vi "Find Scalar Group.vi"(8 "error in (no error)":errorcluster, 10 "Group Name":string, 11 "FPGA Addon refnum in":T1 format="%.0x") -> (0 "error out":errorcluster, 1 "Found ?":bool, 2 "Group Scalar Data":T2 {"Scalar Section ref" format="%.0x"; "Group Section ref" format="%.0x"; "Group Scalar Registers"."Data Type" format="%.0x"}, 3 "FPGA Addon refnum out":T1=18446744073709551615 format="%.0x")   [LabVIEW 2018, in "Scripting API.lvlib"]
uses:
  Scripting API.lvlib
  <vilib>/NI Veristand/Custom Device API/Custom Device Item Ref.ctl
  TypeDefs/Group Scalar Data.ctl
  Addon/Addon Shared/Types/Register Information.ctl
  Addon/Addon Shared/Types/Data Type.ctl
  Addon/Addon Shared/Types/FG Action.ctl
  Addon/Addon Shared/SubVIs/Constants.vi
  <vilib>/NI/NI VeriStand Advanced SysDef API/_SubVIs/SysDef.Search.GUID.vi
  <vilib>/NI/NI VeriStand Advanced SysDef API/SysDef API/SysDef.Property.Get.vi
  <vilib>/NI/NI VeriStand Advanced SysDef API/_SubVIs/SysDef.Property.Get.Variant.vi
  <vilib>/NI/NI VeriStand Advanced SysDef API/SysDef API/SysDef.Property.Set.vi
  <vilib>/NI/NI VeriStand Advanced SysDef API/_SubVIs/SysDef.Property.Set.Variant.vi
  <vilib>/NI/NI VeriStand Advanced SysDef API/_SubVIs/SysDef.Search.Name.vi
  <vilib>/NI/NI VeriStand Advanced SysDef API/SysDef API/Advanced System Definition.lvlib
  Addon/Addon Shared/FPGA Addon Shared.lvlib
  <vilib>/NI Veristand/Custom Device API/Custom Device API.lvlib
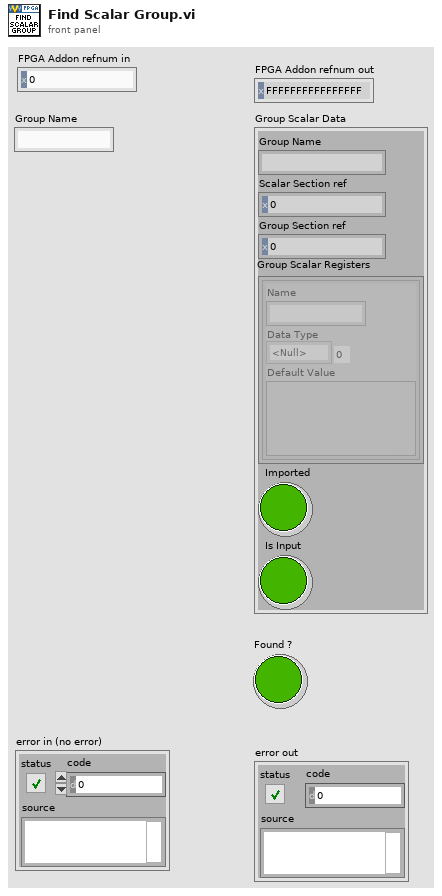
[diagram p1: front panel]
types:
  T1 = typedef "Custom Device API.lvlib/Custom Device Item Ref.ctl" = u64
  T2 = typedef "Scripting API.lvlib/Group Scalar Data.ctl" = cluster{"Group Name":string, "Scalar Section ref":T1, "Group Section ref":T1, "Group Scalar Registers":T3[], "Imported":bool, "Is Input":bool}
  T3 = typedef "FPGA Addon Shared.lvlib/Register Information.ctl" = cluster{"Name":string, "Data Type":T4, "Default Value":variant}
  T4 = typedef "FPGA Addon Shared.lvlib/Data Type.ctl" = enum8{"<Null>", "I8", "I16", "I32", "I64", "U8", "U16", "U32", "U64", "SGL", "Boolean", "Analog PWM In Settings", "Analog PWM In", "Digital PWM In Settings", "Digital PWM In", "Digital PWM Out", "Sine Out", "FXP+/-24.5", "FXP+/-16.5", "FXP+/-32.8", "FXP+/-64.32", "FXP+/-16.7", "FXP+/-20.5", "FXP+/-27.5", "FXP+/-32.16", "FXP+16.3", "FXP+18.3", "Digital Static In", "Digital Static Out", "Digital Static In Settings", "Digital WSS Out", "Quad Encoder Settings", "Quad Encoder In", "Group"}
  T5 = typedef "FPGA Addon Shared.lvlib/FG Action.ctl" = enum8{"GET", "SET"}
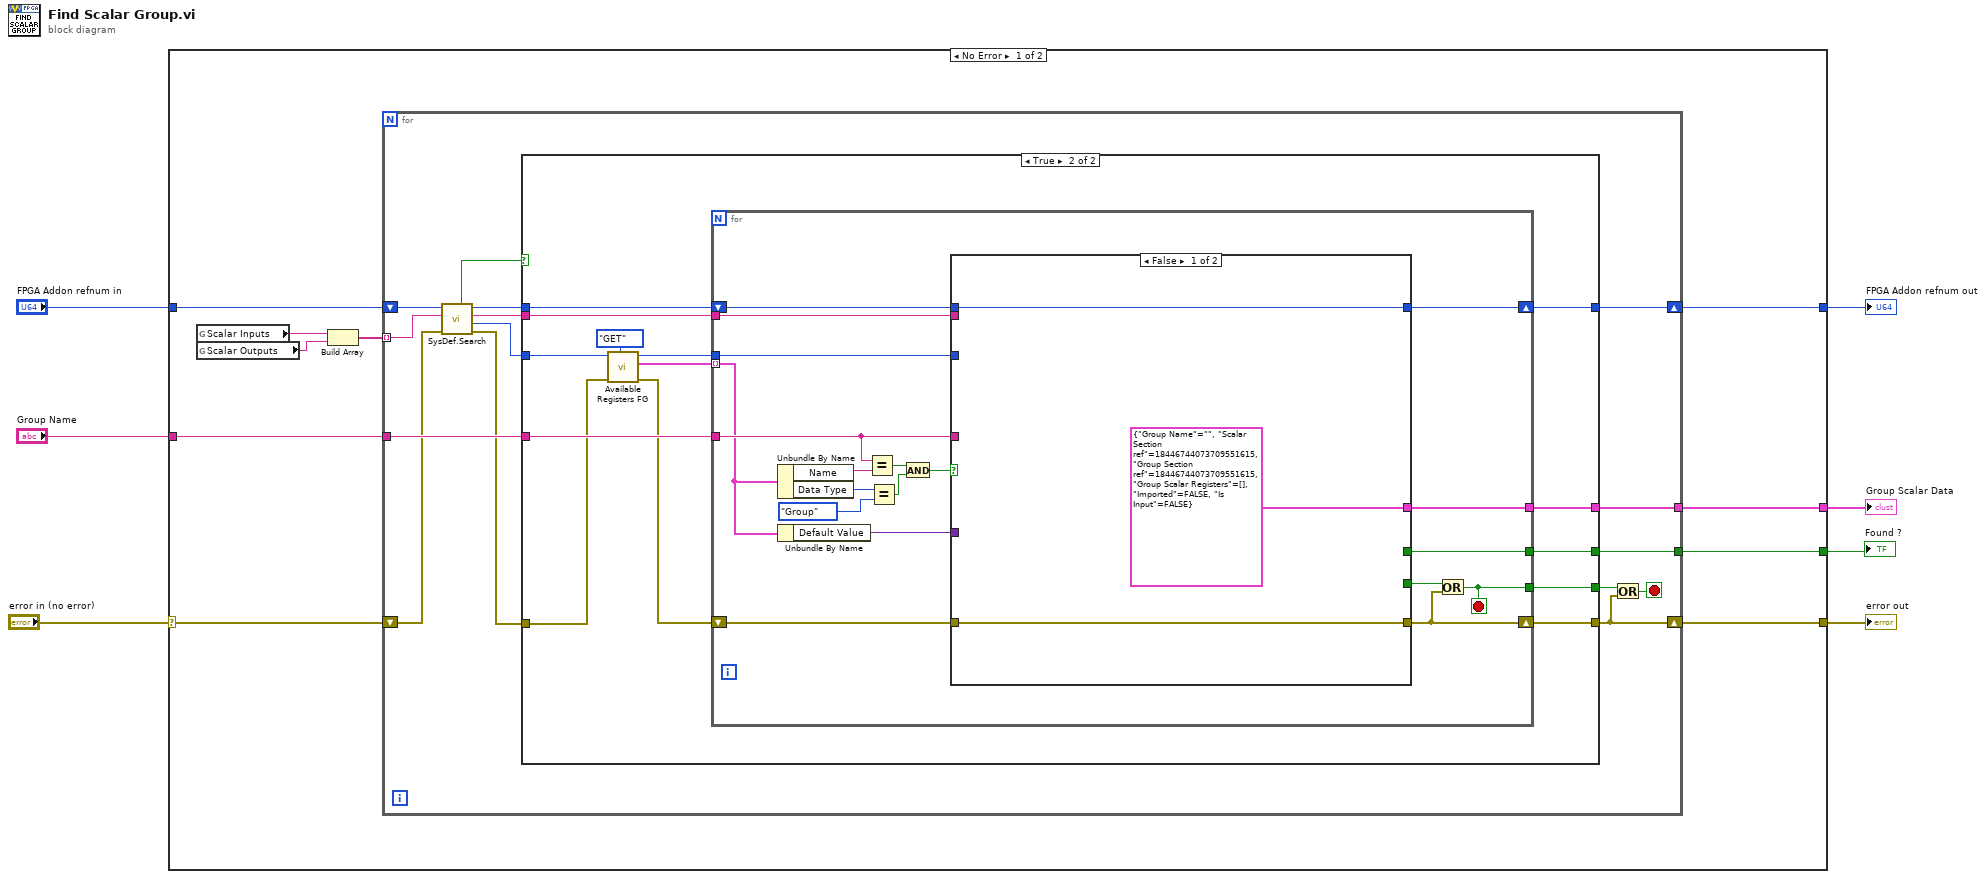
[diagram p0: block diagram]
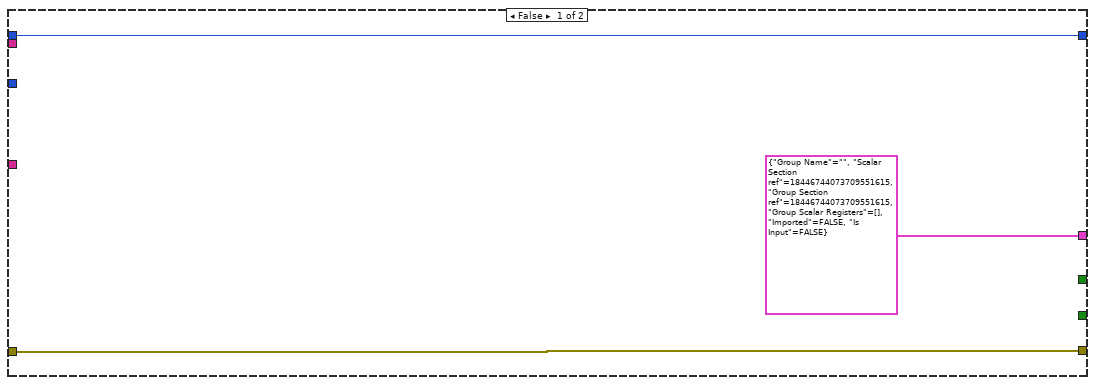
[diagram p2: hidden frame]
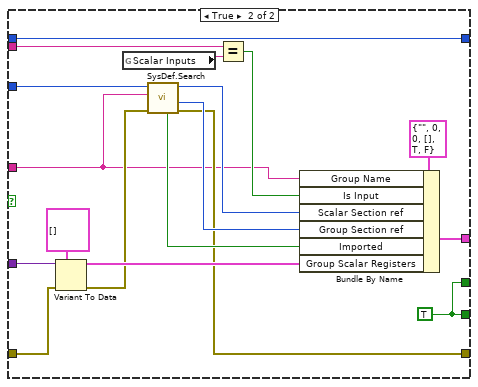
[diagram p3: hidden frame]
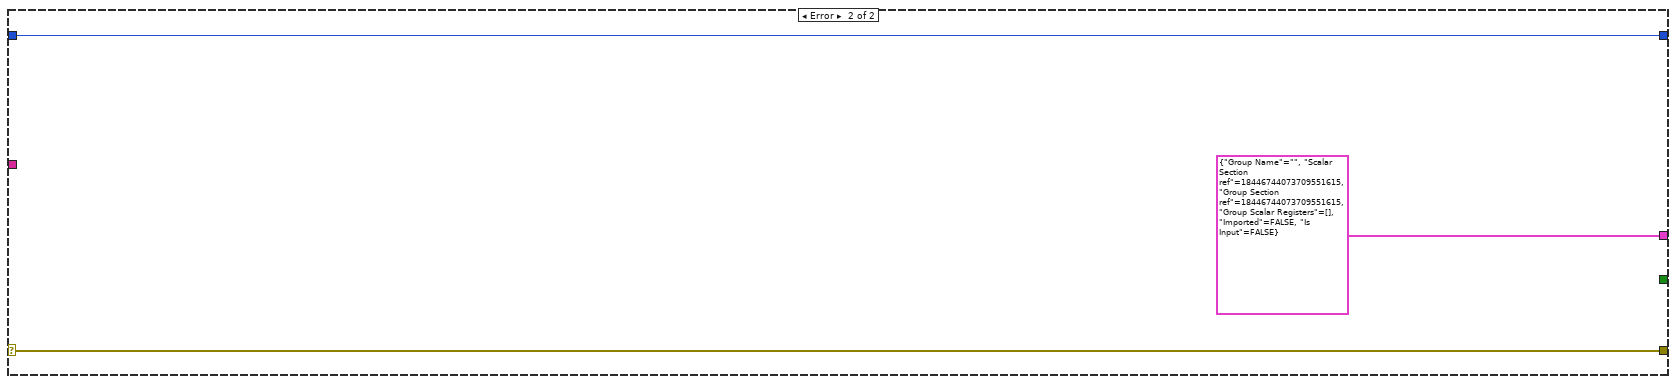
[diagram p4: hidden frame]
diagram:
  n1 = case shown="No Error" "error in (no error)" {
    selector: "error in (no error)" -> [w12 w91]
    tunnel: "Group Name" -> [w17 _]
    tunnel: "FPGA Addon refnum in" -> [w13 w89]
    tunnel: [w11 w91] -> w4
    tunnel: [w10 T2 {"Group Name"="", "Scalar Section ref"=18446744073709551615, "Group Section ref"=18446744073709551615, "Group Scalar Registers"=[], "Imported"=FALSE, "Is Input"=FALSE}] -> w3
    tunnel: [w9 w89] -> w2
    tunnel: [w8 _] -> w1
    frame No Error {
      n2 = global read "Constants.vi" "Scalar Inputs"() -> (w15:string)
      n3 = global read "Constants.vi" "Scalar Outputs"() -> (w14:string)
      n4 = Build Array(w15, w14) -> (w16:string[])
      n5 = for {
        tunnel: w16 -> [w18] mode=indexing
        tunnel: w17 -> [w29]
        shift-right: [w26] -> w9
        shift-left: w13 -> [w31]
        tunnel: [w25] -> w10
        shift-right: [w22] -> w11
        shift-left: w12 -> [w24]
        tunnel: [w19] -> w8
        stop <- w20 stop-if-true
        n6 = call-poly <vilib>:"SysDef.Search.vi"("error in (no error)"=w24, "GUID"=w18, "nodeID"=w31) -> ("error out"=w23:errorcluster, "Value out"=w30:u64, "nodeID out"=w27:u64, "Found?"=w28:bool)  [unwired: 5 in]
        n7 = case shown="True" w28 {
          tunnel: w30 -> [_ w47]
          tunnel: w29 -> [_ w46]
          tunnel: w27 -> [w34 w43]
          tunnel: [w34 w42] -> w26
          tunnel: [T2 {"Group Name"="", "Scalar Section ref"=18446744073709551615, "Group Section ref"=18446744073709551615, "Group Scalar Registers"=[], "Imported"=FALSE, "Is Input"=FALSE} w41] -> w25
          tunnel: w23 -> [w33 w40]
          tunnel: [_ w38] -> w21
          tunnel: [w33 w37] -> w22
          tunnel: [_ w36] -> w19
          tunnel: w18 -> [_ w35]
          frame False {
          }
          frame True {
            n8 = call "Available Registers FG.vi"("Action"=FG_Action."GET", "error in (no error)"=w40, "Item Ref"=w47) -> ("error out"=w39:errorcluster, "Available Registers"=w44:T3[], "Item Ref out"=w45:T1)  [unwired: 6 in]
            n9 = for {
              tunnel: w44 -> [w58] mode=indexing
              tunnel: w46 -> [w59]
              tunnel: w45 -> [w64]
              shift-right: [w56] -> w42
              shift-left: w43 -> [w63]
              tunnel: [w55] -> w41
              shift-right: [w51] -> w37
              shift-left: w39 -> [w54]
              tunnel: [w53] -> w38
              tunnel: [w50] -> w36
              tunnel: w35 -> [w49]
              stop <- w53 stop-if-true
              n10 = Unbundle By Name(w58) -> ("Name"=w60:string, "Data Type"=w62:T4)
              n11 = Unbundle By Name(w58) -> ("Default Value"=w57:variant)
              n12 = Equal?(x=w59, y=w60) -> (x = y?=w67:bool)
              n13 = Equal?(x=w62, y=Data_Type."Group" ("x")) -> (x = y?=w66:bool)
              n14 = And(x=w67, y=w66) -> (x .and. y?=w65:bool)
              n15 = case shown="False" w65 {
                tunnel: w64 -> [_ w88]
                tunnel: w63 -> [w70 w81]
                tunnel: w59 -> [_ w71]
                tunnel: w57 -> [_ w84]
                tunnel: [w70 w81] -> w56
                tunnel: [T2 {"Group Name"="", "Scalar Section ref"=18446744073709551615, "Group Section ref"=18446744073709551615, "Group Scalar Registers"=[], "Imported"=FALSE, "Is Input"=FALSE} w80] -> w55
                tunnel: w54 -> [w68 w78]
                tunnel: [w68 w79] -> w51
                tunnel: [_ w75] -> w52
                tunnel: [_ w75] -> w50
                tunnel: w49 -> [_ w74]
                frame False {
                }
                frame True {
                  w75 = TRUE
                  n16 = Variant To Data(error in=w78, type=T3[] [], Variant=w84) -> (data=w82:T3[], error out=w77:errorcluster)
                  n17 = global read "Constants.vi" "Scalar Inputs"() -> (w73:string)
                  n18 = call-poly <vilib>:"SysDef.Search.vi"("error in (no error)"=w77, "Name"=w71, "nodeID"=w88) -> ("error out"=w79:errorcluster, "Value out"=w86:u64, "nodeID out"=w85:u64, "Found?"=w87:bool)  [unwired: 5 in]
                  n19 = Equal?(x=w74, y=w73) -> (x = y?=w72:bool)
                  n20 = Bundle By Name(cluster=T2 {"Group Name"="", "Scalar Section ref"=0, "Group Section ref"=0, "Group Scalar Registers"=[], "Imported"=TRUE, "Is Input"=FALSE}, "Group Name"=w71, "Is Input"=w72, "Scalar Section ref"=w85, "Group Section ref"=w86, "Imported"=w87, "Group Scalar Registers"=w82) -> (w80:T2)
                }
              }
              n21 = Or(x=w52, y=w51) -> (x .or. y?=w53:bool)
            }
          }
        }
        n22 = Or(x=w21, y=w22) -> (x .or. y?=w20:bool)
      }
    }
    frame Error {
    }
  }
  "error out" <- w4
  "Group Scalar Data" <- w3
  "FPGA Addon refnum out" <- w2
  "Found ?" <- w1
